vi "Write configuration.vi"(8 "error in":errorcluster, 10 "configuration":refnum<class "NISE_CEF_serializable configuration.lvclass">, 11 "Bus in":refnum<class "Bus.lvclass">) -> (0 "error out":errorcluster, 3 "Bus out":refnum<class "Bus.lvclass">)   [LabVIEW 2014, in "Bus.lvclass"]
uses:
  Bus.lvclass
  <vilib>/NI/Configuration Framework/serializable configuration/NISE_CEF_serializable configuration.lvclass
  Bus Configuration/Bus Configuration.lvclass
  Bus.lvclass/Bus.ctl
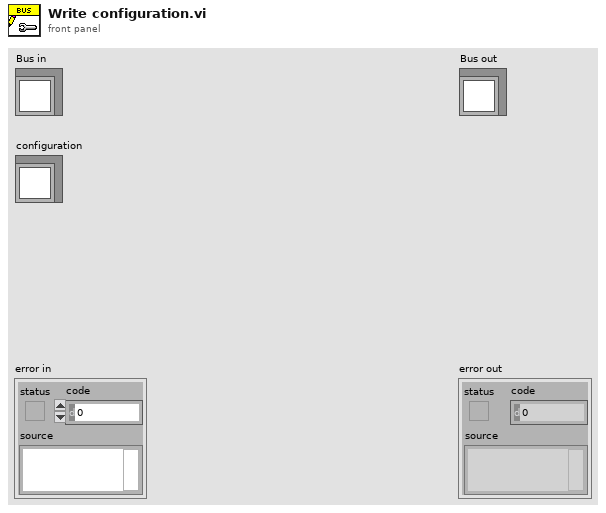
[diagram p1: front panel]
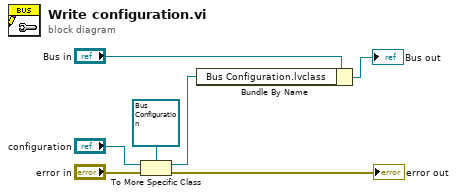
[diagram p0: block diagram]
diagram:
  n1 = To More Specific Class(target class=refnum<class "Bus Configuration.lvclass"> refnum ("Bus Configuration.lvclass"), reference="configuration", error in="error in") -> (specific class reference=w1:refnum<class "Bus Configuration.lvclass">, error out=→"error out":errorcluster)
  n2 = Bundle By Name(cluster="Bus in", "Bus Configuration.lvclass"=w1) -> (→"Bus out":refnum<class "Bus.lvclass">)
